vi "Shutdowncase.vi"(8 "error in (no error)":errorcluster, 10 "Boolean":bool, 11 "Data Cluster":T1 {"Type" items=["Hot Water", "Coffe", "Latte"]; "Chamber" scale=0.0..60.0; "Dispenser" scale=0.0..60.0}) -> (0 "error out":errorcluster, 3 "output cluster":T1={"Cup"=FALSE, "Type"=0, "Carafe"=FALSE, "Bean Level"=0, "Water Level"=0, "Milk Level"=0, "Low Bean"=FALSE, "Low Milk"=FALSE, "Chamber"=1, "Dispenser"=1, "Low Water"=FALSE, "Elapsed Time"=0.0, "Purging"=FALSE, "Heating"=FALSE, "Grinding"=FALSE, "Brewing"=FALSE, "Dispensing"=FALSE, "Total Cups"=0, "Power"=FALSE, "Timer"={"Relative time"=0.0, "Initial Time"=0.0, "Set Timer"=0, "Start/Stop"=FALSE, "Pause/Resume"=FALSE}, "Path"=path "", "Shutdown"=FALSE} {"Type" items=["Hot Water", "Coffe", "Latte"]; "Chamber" scale=0.0..60.0; "Dispenser" scale=0.0..60.0})   [LabVIEW 2020]
uses:
  Typedef/DataCluster.ctl
  Strict Type Def/LowBean.ctl
  Strict Type Def/LowMilk.ctl
  Strict Type Def/Chamber.ctl
  Strict Type Def/Dispenser.ctl
  Strict Type Def/Low Water.ctl
  Strict Type Def/Purging.ctl
  Strict Type Def/Heating.ctl
  Strict Type Def/Grinding.ctl
  Strict Type Def/Brewing.ctl
  Strict Type Def/Dispensing.ctl
  Typedef/TimeCluster.ctl
  Typedef/QueueOperation.ctl
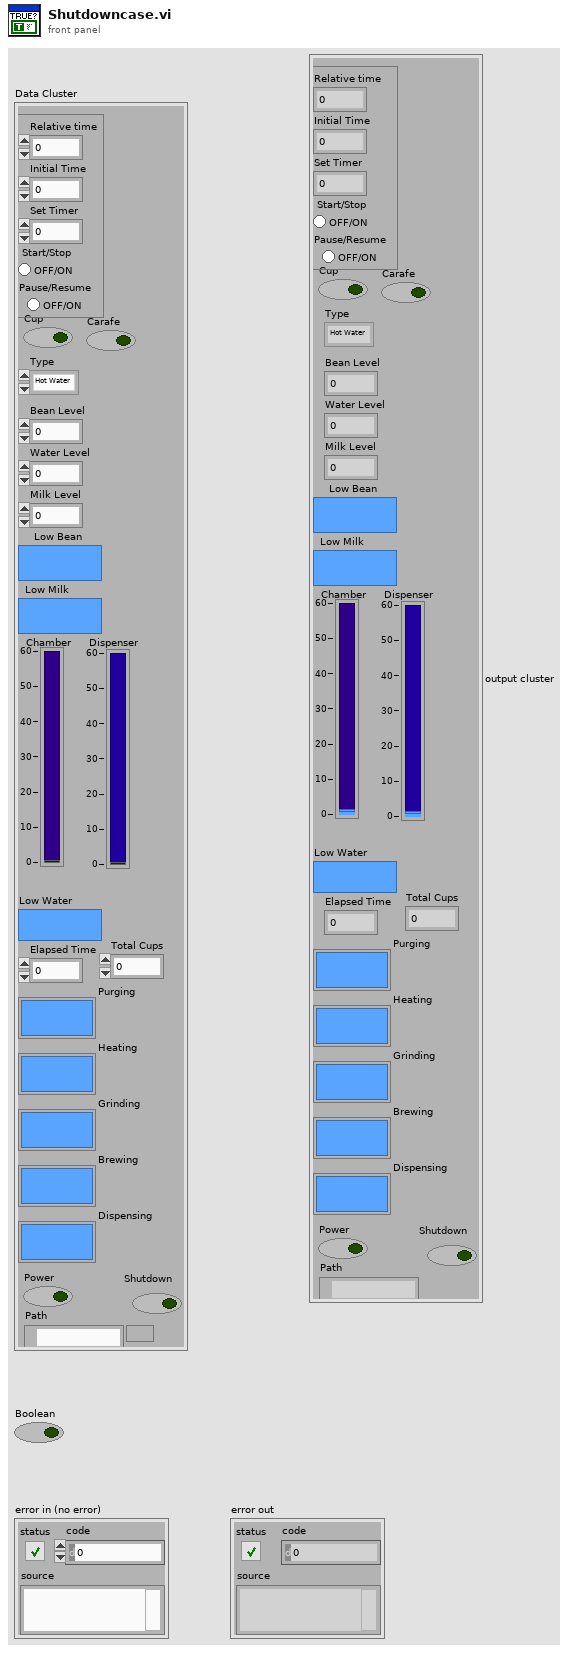
[diagram p1: front panel]
types:
  T1 = typedef "DataCluster.ctl" = cluster{"Cup":bool, "Type":i32, "Carafe":bool, "Bean Level":i32, "Water Level":i32, "Milk Level":i32, "Low Bean":T2, "Low Milk":T3, "Chamber":T4, "Dispenser":T5, "Low Water":T6, "Elapsed Time":dbl, "Purging":T7, "Heating":T8, "Grinding":T9, "Brewing":T10, "Dispensing":T11, "Total Cups":i32, "Power":bool, "Timer":T12, "Path":path, "Shutdown":bool}
  T2 = typedef "LowBean.ctl" = bool
  T3 = typedef "LowMilk.ctl" = bool
  T4 = typedef "Chamber.ctl" = u8
  T5 = typedef "Dispenser.ctl" = u8
  T6 = typedef "Low Water.ctl" = bool
  T7 = typedef "Purging.ctl" = bool
  T8 = typedef "Heating.ctl" = bool
  T9 = typedef "Grinding.ctl" = bool
  T10 = typedef "Brewing.ctl" = bool
  T11 = typedef "Dispensing.ctl" = bool
  T12 = typedef "TimeCluster.ctl" = cluster{"Relative time":dbl, "Initial Time":dbl, "Set Timer":i32, "Start/Stop":bool, "Pause/Resume":bool}
  T13 = typedef "QueueOperation.ctl" = enum16{"Create", "Enqueue", "Dequeue", "Flush", "Close"}
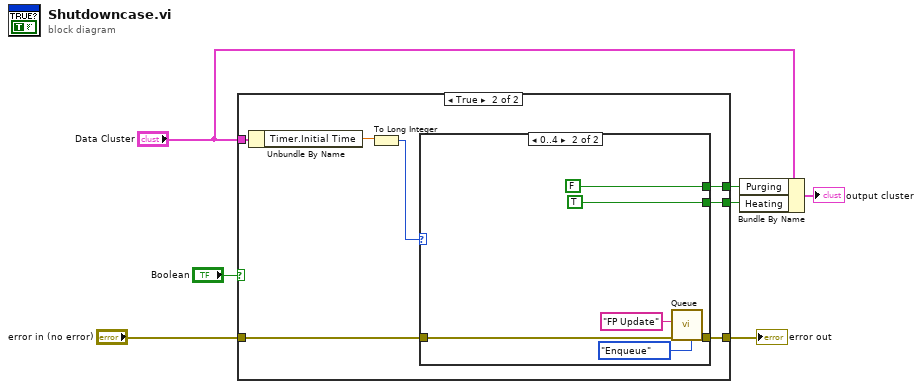
[diagram p0: block diagram]
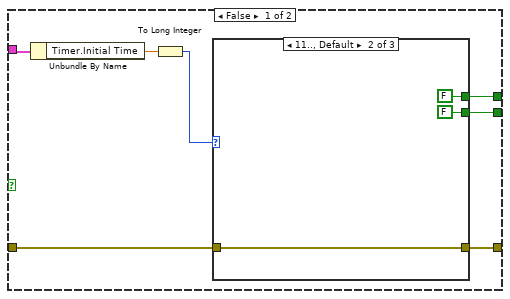
[diagram p2: hidden frame]
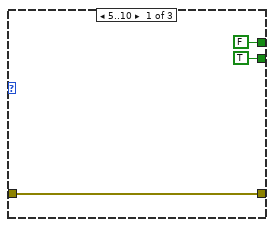
[diagram p3: hidden frame]
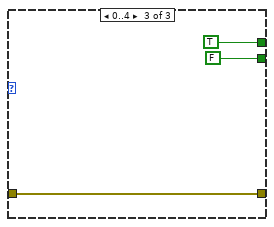
[diagram p4: hidden frame]
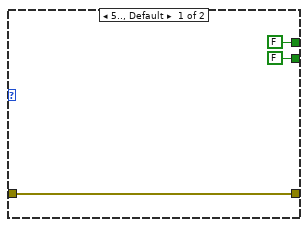
[diagram p5: hidden frame]
diagram:
  n1 = case shown="True" "Boolean" {
    tunnel: [w12 w30] -> w5
    tunnel: "error in (no error)" -> [w11 w29]
    tunnel: "Data Cluster" -> [w14 w28]
    tunnel: [w8 w25] -> w3
    tunnel: [w9 w24] -> w2
    frame False {
      n2 = Unbundle By Name(w14) -> ("Timer.Initial Time"=w13:dbl)
      n3 = To Long Integer(number=w13) -> (32bit integer=w10:i32)
      n4 = case shown="11.., Default" w10 {
        tunnel: [w15 w18 w23] -> w12
        tunnel: w11 -> [w15 w18 w23]
        tunnel: [T7 FALSE ("Purging") T7 FALSE ("Purging") T7 TRUE ("Purging")] -> w9
        tunnel: [T8 TRUE ("Heating") T8 FALSE ("Heating") T8 FALSE ("Heating")] -> w8
        frame 5..10 {
        }
        frame 11.., Default {
        }
        frame 0..4 {
        }
      }
    }
    frame True {
      n5 = Unbundle By Name(w28) -> ("Timer.Initial Time"=w27:dbl)
      n6 = To Long Integer(number=w27) -> (32bit integer=w26:i32)
      n7 = case shown="0..4" w26 {
        tunnel: [w31 w39] -> w30
        tunnel: w29 -> [w31 w38]
        tunnel: [T8 FALSE ("Heating") T8 TRUE ("Heating")] -> w25
        tunnel: [T7 FALSE ("Purging") T7 FALSE ("Purging")] -> w24
        frame 5.., Default {
        }
        frame 0..4 {
          n8 = call "Queue.vi"("Enum"=QueueOperation."Enqueue", "error in (no error)"=w38, "Enqueue Element"="FP Update") -> ("error out"=w39:errorcluster)  [unwired: 6 in, 2 out]
        }
      }
    }
  }
  "error out" <- w5
  n9 = Bundle By Name(cluster="Data Cluster", "Purging"=w2, "Heating"=w3) -> (→"output cluster":T1)
